vi "Write DMA FIFO.vi"(8 "error in (no error)":errorcluster, 10 "FIU SPI Commands":u64[](array[numeric]), 11 "DMA FIFO Ref in":refnum<k20>) -> (0 "error out":errorcluster)   [LabVIEW 2014, in "SLSC configuration Engine.lvlib"]
uses:
  SLSC configuration Engine.lvlib
  <vilib>/Utility/error.llb/Error Cluster From Error Code.vi
  <vilib>/rvi/errors/niLvFpgaAdjustHostInterfaceError.vi
  <vilib>/rvi/interface/nirviMethod/nirviMethod.xnode
  <vilib>/FPGAPlugInAG/Dynamic/niLvFpga_WriteFifo_Dynamic.vi
  <vilib>/rvi/errors/niLvFpgaMergeErrorWithErrorCode.vi
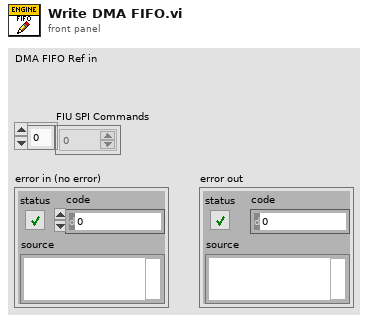
[diagram p1: front panel]
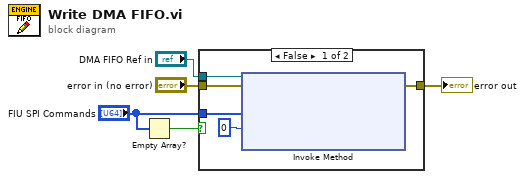
[diagram p0: block diagram]
diagram:
  n1 = Empty Array?(array="FIU SPI Commands") -> (empty?=w2:bool)
  n2 = case shown="False" w2 {
    tunnel: "DMA FIFO Ref in" -> [w10 _]
    tunnel: "error in (no error)" -> [w8 w11]
    tunnel: [w7 w11] -> w3
    tunnel: "FIU SPI Commands" -> [w6 _]
    frame False {
      n3 = xnode "Invoke Method"("FPGA VI Reference In"=w10, "error in"=w8, "Data"=w6, "Timeout (ms)"=0) -> ("error out"=w7:errorcluster)  [unwired: 2 out]
    }
    frame True {
    }
  }
  "error out" <- w3
